vi "save_TRABS.vi"(6 "TRABS":dbl[][](array[numeric]), 8 "error in (no error)":errorcluster, 9 "filename":string, 10 "type":string, 11 "dict of HIS IN":variant) -> (0 "error out":errorcluster, 3 "dict of HIS OUT":variant)   [LabVIEW 2015]
uses:
  cluster_template.ctl
  Classes/DATA/HIS/HIS.lvclass
  Classes/DATA/DATA.lvclass/DATA.ctl
  <vilib>/Utility/file.llb/Write Delimited Spreadsheet (DBL).vi
  Classes/DATA/DATA.lvclass
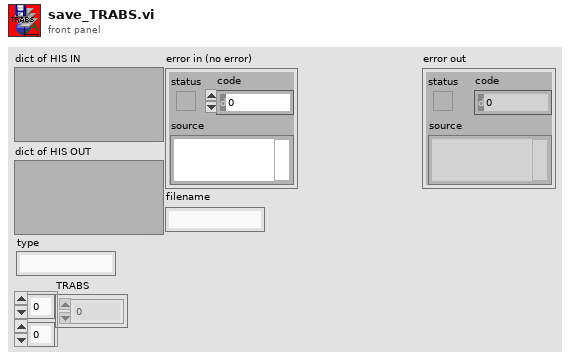
[diagram p1: front panel]
types:
  T1 = typedef "cluster_template.ctl" = cluster{"HIS.lvclass":refnum<class "HIS.lvclass">, "selector":refnum<vi>, "HIS graph":refnum<vi>, "DAT graph":refnum<vi>, "path":refnum<vi>, "path MAIN":refnum<vi>, "#":refnum<vi>, "unsel Graph":refnum<vi>, "DATgraph":refnum<vi>}
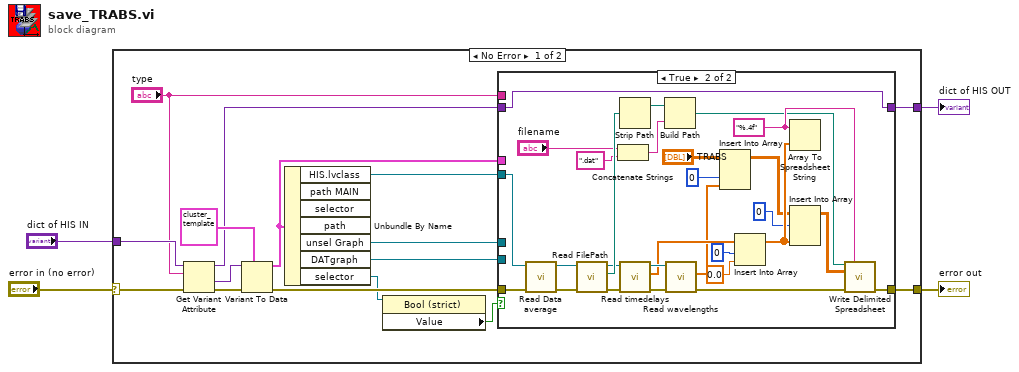
[diagram p0: block diagram]
diagram:
  n1 = case shown="No Error" "error in (no error)" {
    selector: "error in (no error)" -> [w19 w52]
    tunnel: "dict of HIS IN" -> [w20 w51]
    tunnel: [w14 w51] -> w3
    tunnel: [w5 w52] -> w2
    frame No Error {
      n2 = Get Variant Attribute(Variant=w20, name="type", error in=w19) -> (duplicate Variant=w13:variant, value=w18:variant, error out=w17:errorcluster)  [unwired: 1 in, 1 out]
      n3 = Variant To Data(error in=w17, type=T1 {"HIS.lvclass"=refnum, "selector"=refnum, "HIS graph"=refnum, "DAT graph"=refnum, "path"=refnum, "path MAIN"=refnum, "#"=refnum, "unsel Graph"=refnum, "DATgraph"=refnum} ("output cluster"), Variant=w18) -> (data=w15:T1, error out=w10:errorcluster)
      n4 = Unbundle By Name(w15) -> ("HIS.lvclass"=w9:refnum<class "HIS.lvclass">, "unsel Graph"=w11:refnum<vi>, "DATgraph"=w8:refnum<vi>, "selector"=w7:refnum<vi>)  [unwired: 3 out]
      n5 = property class="Bool (strict)"(reference=w7) -> ("Value"=w6:bool)  [unwired: 1 in, 2 out]
      n6 = case shown="True" w6 {
        tunnel: w15 -> [_ _]
        tunnel: [w22 w48] -> w14
        tunnel: w13 -> [w22 w48]
        tunnel: "type" -> [_ _]
        tunnel: w11 -> [_ _]
        tunnel: w10 -> [w21 w27]
        tunnel: w9 -> [_ w28]
        tunnel: w8 -> [_ _]
        tunnel: [w21 w30] -> w5
        frame False {
        }
        frame True {
          w32 = "%.4f" ("format string")
          n7 = call "Read Data average.vi"("error in (no error)"=w27, "DATA in"=w28) -> ("error out"=w50:errorcluster, "DATA out"=w49:refnum<class "HIS.lvclass">)  [unwired: 7 in, 1 out]
          n8 = call "Read FilePath.vi"("error in (no error)"=w50, "DATA in"=w49) -> ("error out"=w42:errorcluster, "FilePath"=w46:path, "DATA out"=w41:refnum<class "HIS.lvclass">)  [unwired: 7 in]
          n9 = Concatenate Strings("filename", ".dat" ("string")) -> (w43:string)
          n10 = Strip Path(path=w46) -> (stripped path=w47:path)  [unwired: 1 out]
          n11 = call "Read timedelays.vi"("error in (no error)"=w42, "DATA in"=w41) -> ("error out"=w40:errorcluster, "timedelays"=w38:dbl[], "DATA out"=w39:refnum<class "HIS.lvclass">)  [unwired: 7 in]
          n12 = Build Path(base path=w47, name or relative path=w43) -> (appended path=w29:path)
          n13 = call "Read wavelengths.vi"("error in (no error)"=w40, "DATA in"=w39) -> ("error out"=w31:errorcluster, "wavelengths"=w35:dbl[])  [unwired: 7 in, 1 out]
          n14 = Insert Into Array(array="TRABS", index (col)=0 ("disabled index (col)"), new element=w35) -> (w25:dbl[][])  [unwired: 1 in]
          n15 = Insert Into Array(array=w38, index=0, new element=0.0 ("new element/subarray")) -> (w34:dbl[])
          n16 = Array To Spreadsheet String(array=w34, 3:w32) -> ()  [unwired: 1 in, 1 out]
          n17 = Insert Into Array(array=w25, index (row)=0, new element=w34) -> (w33:dbl[][])  [unwired: 1 in]
          n18 = call-poly <vilib>:"Write Delimited Spreadsheet.vi"("file path (dialog if empty)"=w29, "format (%.3f)"=w32, "2D data"=w33, "error in (no error)"=w31) -> ("error out"=w30:errorcluster)  [unwired: 10 in, 1 out]
        }
      }
    }
    frame Error {
    }
  }
  "dict of HIS OUT" <- w3
  "error out" <- w2
